vi "Read Bounds.vi"(8 "error in (no error)":errorcluster, 11 "window in":refnum<class "window.lvclass">) -> (0 "error out":errorcluster, 2 "Bounds":T1, 3 "window out":refnum<class "window.lvclass">)   [LabVIEW 2013, in "frontPanelObjects.lvlib" / "window.lvclass"]
uses:
  window.lvclass
  <vilib>/Utility/miscctls.llb/LVBoundsTypeDef.ctl
  window.lvclass/window.ctl
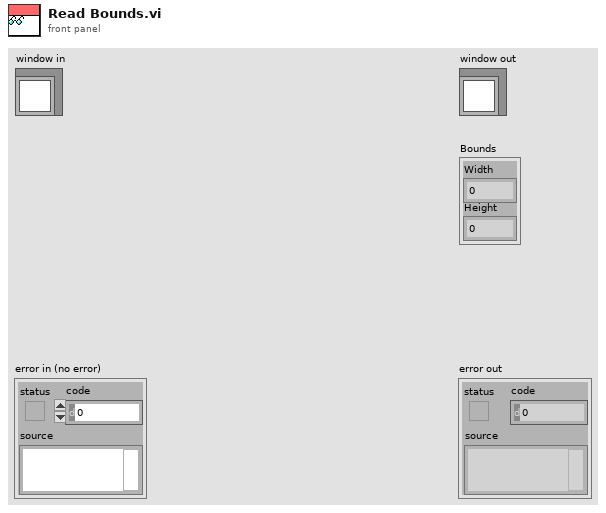
[diagram p1: front panel]
types:
  T1 = typedef "LVBoundsTypeDef.ctl" = cluster{"Width":u32, "Height":u32}
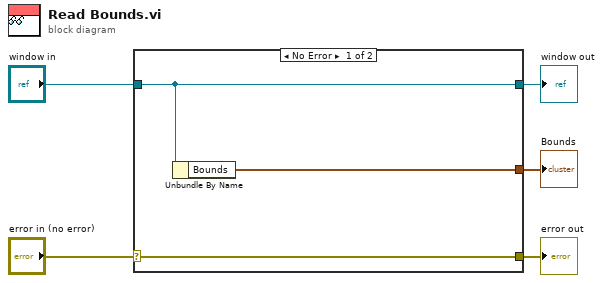
[diagram p0: block diagram]
diagram:
  n1 = case shown="No Error" "error in (no error)" {
    selector: "error in (no error)" -> [w8 w9]
    tunnel: [w8 w9] -> w4
    tunnel: [w7 w10] -> w2
    tunnel: "window in" -> [w7 w10]
    tunnel: [w6 _] -> w1
    frame No Error {
      n2 = Unbundle By Name(w7) -> ("Bounds"=w6:T1)
    }
    frame Error {
    }
  }
  "error out" <- w4
  "window out" <- w2
  "Bounds" <- w1
